vi "Find Neighbours.vi"(6 "#":i32=33, 7 "Add Start Point?":bool, 10 "Points In":i32[][](array[numeric]), 11 "XY":i32[](array[numeric])) -> (2 "Points out":i32[][](array[numeric]), 3 "Filtered":i32[][](array[numeric]))   [LabVIEW 2021, in "lv_icon.lvlib"]
doc: "Find neighbour pixels with the same color. \nThis algorithm only considers horizontal and vertical pixels."
uses:
  <vilib>/LabVIEW Icon API/lv_icon/lv_icon.lvlib
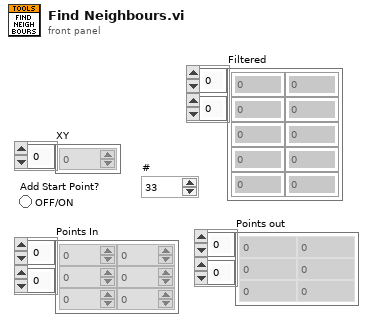
[diagram p1: front panel]
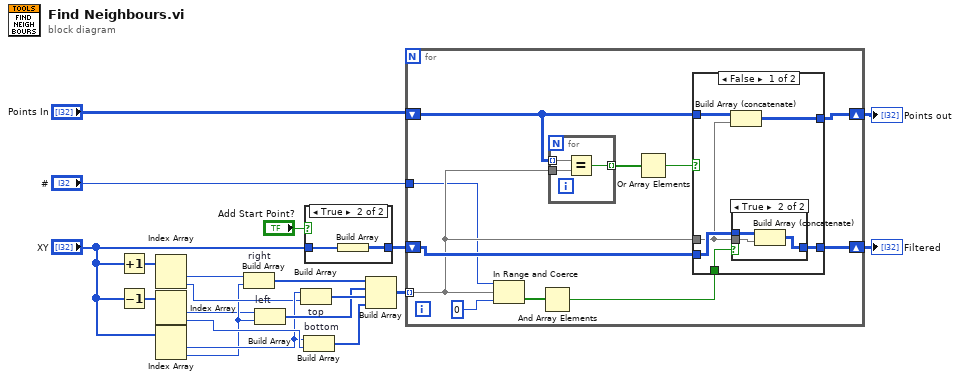
[diagram p0: block diagram]
diagram:
  n1 = Increment(x="XY") -> (x+1=w9:i32[])
  n2 = Decrement(x="XY") -> (x-1=w10:i32[])
  n3 = Index Array(array=w9) -> (element #1=w11:i32, element #2=w14:i32)  [unwired: 2 in]
  n4 = Index Array(array=w10) -> (element #1=w12:i32, element #2=w16:i32)  [unwired: 2 in]
  n5 = Index Array(array="XY") -> (element #1=w15:i32, element #2=w13:i32)  [unwired: 2 in]
  n6 = Build Array "right"(w11, w13) -> (w17:i32[])
  n7 = Build Array "left"(w12, w13) -> (w18:i32[])
  n8 = Build Array "top"(w15, w14) -> (w19:i32[])
  n9 = Build Array "bottom"(w15, w16) -> (w20:i32[])
  n10 = case shown="True" "Add Start Point?" {
    tunnel: [_ w22] -> w6
    tunnel: "XY" -> [_ w21]
    frame False {
    }
    frame True {
      n11 = Build Array(w21) -> (w22:i32[][])
    }
  }
  n12 = Build Array(w17, w18, w19, w20) -> (w8:i32[][])
  n13 = for {
    tunnel: w8 -> [w28] mode=indexing
    shift-right: [w30] -> w7
    shift-left: w6 -> [w29]
    shift-right: [w25] -> w2
    shift-left: "Points In" -> [w24]
    tunnel: "#" -> [w23]
    n14 = In Range and Coerce(upper limit=w23, x=w28, lower limit=0) -> (In Range?=w32:bool[])  [unwired: 1 out]
    n15 = And Array Elements(Boolean array=w32) -> (logical AND=w31:bool)
    n16 = for {
      tunnel: w24 -> [w48] mode=indexing
      tunnel: w28 -> [w47]
      tunnel: [w46] -> w27 mode=indexing
      n17 = Equal?(x=w48, y=w47) -> (x = y?=w46:bool)
    }
    n18 = Or Array Elements(Boolean array=w27) -> (logical OR=w26:bool)
    n19 = case shown="False" w26 {
      tunnel: w31 -> [w34 _]
      tunnel: [w35 w45] -> w30
      tunnel: w29 -> [w39 w45]
      tunnel: w28 -> [w37 _]
      tunnel: w24 -> [w38 w44]
      tunnel: [w36 w44] -> w25
      frame False {
        n20 = Build Array (concatenate)(w38, w37) -> (w36:i32[][])
        n21 = case shown="True" w34 {
          tunnel: w39 -> [w40 w43]
          tunnel: w37 -> [_ w42]
          tunnel: [w40 w41] -> w35
          frame False {
          }
          frame True {
            n22 = Build Array (concatenate)(w43, w42) -> (w41:i32[][])
          }
        }
      }
      frame True {
      }
    }
  }
  "Filtered" <- w7
  "Points out" <- w2
